vi "Create_Trajectory_Get_Field_Info.vi"(11 "Field Selector":string) -> (2 "value":string, 3 "input cluster":T1)   [LabVIEW 2019]
uses:
  TrajectoryUtils_Field_Info.ctl
  <vilib>/Utility/config.llb/Read Key (String).vi
  <vilib>/Utility/config.llb/Read Key (I32).vi
  <vilib>/Utility/config.llb/Read Key (Double).vi
  <vilib>/Utility/config.llb/NI_LVConfig.lvlib
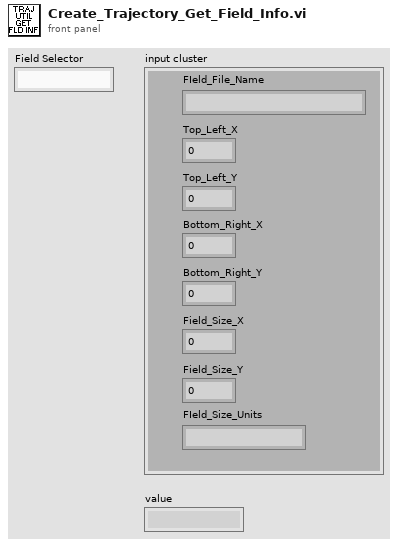
[diagram p1: front panel]
types:
  T1 = typedef "TrajectoryUtils_Field_Info.ctl" = cluster{"FIeld_File_Name":string, "Top_Left_X":i32, "Top_Left_Y":i32, "Bottom_Right_X":i32, "Bottom_Right_Y":i32, "Field_Size_X":dbl, "Field_Size_Y":dbl, "FIeld_Size_Units":string}
  T2 = typedef "NI_LVConfig.lvlib/Config Data RefNum.ctl" = refnum<k1>
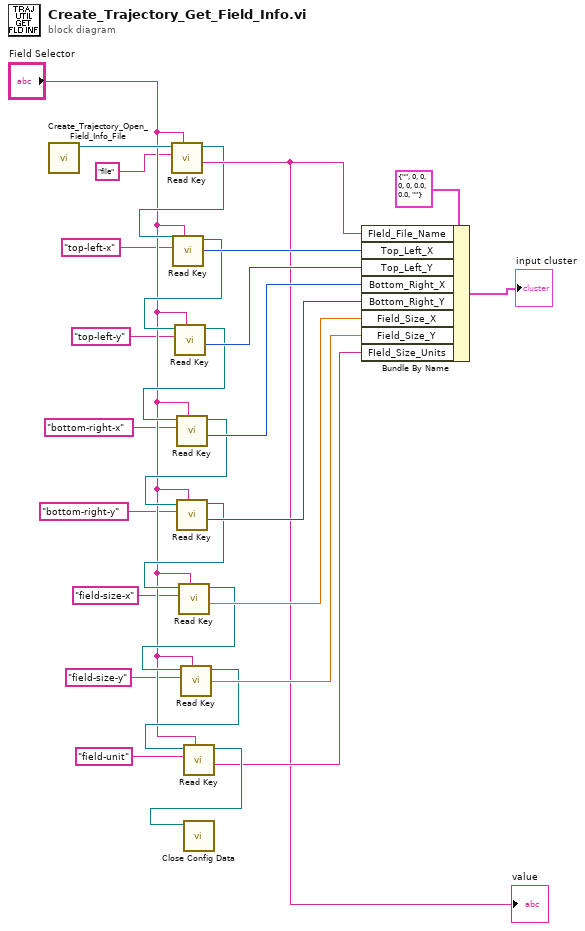
[diagram p0: block diagram]
diagram:
  n1 = call "Create_Trajectory_Open_Field_Info_File.vi"() -> ("Refnum out"=w10:T2)  [unwired: 10 in, 1 out]
  n2 = call-poly <vilib>:"Read Key.vi"("section"="Field Selector", "key"="file", "refnum"=w10) -> ("value"=w19:string, "refnum out"=w11:T2)  [unwired: 5 in, 2 out]
  "value" <- w19
  n3 = call-poly <vilib>:"Read Key.vi"("section"="Field Selector", "key"="top-left-x", "refnum"=w11) -> ("value"=w24:i32, "refnum out"=w12:T2)  [unwired: 5 in, 2 out]
  n4 = call-poly <vilib>:"Read Key.vi"("section"="Field Selector", "key"="top-left-y", "refnum"=w12) -> ("value"=w21:i32, "refnum out"=w13:T2)  [unwired: 5 in, 2 out]
  n5 = call-poly <vilib>:"Read Key.vi"("section"="Field Selector", "key"="bottom-right-x", "refnum"=w13) -> ("value"=w25:i32, "refnum out"=w14:T2)  [unwired: 5 in, 2 out]
  n6 = call-poly <vilib>:"Read Key.vi"("section"="Field Selector", "key"="bottom-right-y", "refnum"=w14) -> ("value"=w22:i32, "refnum out"=w15:T2)  [unwired: 5 in, 2 out]
  n7 = call-poly <vilib>:"Read Key.vi"("section"="Field Selector", "key"="field-size-x", "refnum"=w15) -> ("value"=w23:dbl, "refnum out"=w16:T2)  [unwired: 5 in, 2 out]
  n8 = call-poly <vilib>:"Read Key.vi"("section"="Field Selector", "key"="field-size-y", "refnum"=w16) -> ("value"=w26:dbl, "refnum out"=w17:T2)  [unwired: 5 in, 2 out]
  n9 = call-poly <vilib>:"Read Key.vi"("section"="Field Selector", "key"="field-unit", "refnum"=w17) -> ("value"=w27:string, "refnum out"=w28:T2)  [unwired: 5 in, 2 out]
  n10 = call <vilib>:"Close Config Data.vi"("refnum"=w28) -> ()  [unwired: 9 in, 2 out]
  n11 = Bundle By Name(cluster=T1 {"FIeld_File_Name"="", "Top_Left_X"=0, "Top_Left_Y"=0, "Bottom_Right_X"=0, "Bottom_Right_Y"=0, "Field_Size_X"=0.0, "Field_Size_Y"=0.0, "FIeld_Size_Units"=""} ("input cluster"), "FIeld_File_Name"=w19, "Top_Left_X"=w24, "Top_Left_Y"=w21, "Bottom_Right_X"=w25, "Bottom_Right_Y"=w22, "Field_Size_X"=w23, "Field_Size_Y"=w26, "FIeld_Size_Units"=w27) -> (→"input cluster":T1)
